vi "FGV_volt_flag_G01.vi"(7 "Action":T1, 8 "error in (no error)":errorcluster, 11 "flag in":bool) -> (0 "error out":errorcluster, 3 "flag out":bool)   [LabVIEW 2018]
uses:
  Controls/FGV_voltflag_action.ctl
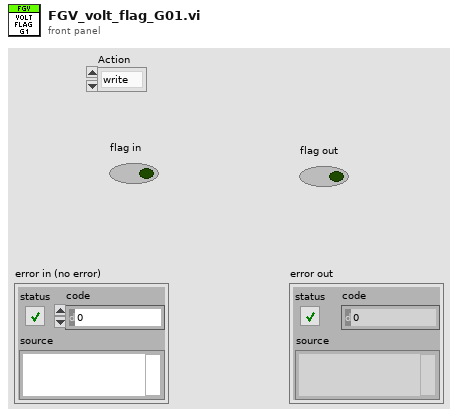
[diagram p1: front panel]
types:
  T1 = typedef "FGV_voltflag_action.ctl" = enum16{"write", "read"}
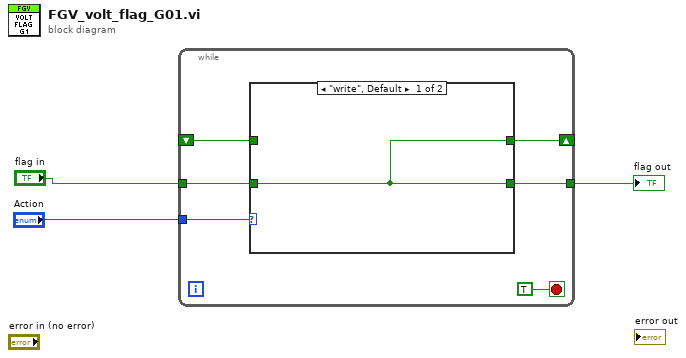
[diagram p0: block diagram]
diagram:
  n1 = while {
    tunnel: "Action" -> [w8]
    shift-right: [w5] -> _
    shift-left: _ -> [w6]
    tunnel: [w7] -> w1
    tunnel: "flag in" -> [w4]
    stop <- TRUE stop-if-true
    n2 = case shown="\"write\", Default" w8 {
      tunnel: [w10 w11] -> w7
      tunnel: w6 -> [_ w11]
      tunnel: [w10 w11] -> w5
      tunnel: w4 -> [w10 _]
      frame "write", Default {
      }
      frame "read" {
      }
    }
  }
  "flag out" <- w1
